vi "communication manager.vi"() -> ()   [LabVIEW 2018]
uses:
  communication-manager/socket REP/socket REP.lvclass
  C:/Users/Denis/Desktop/S4ACS/S4ACS/communication-manager/Socket/Socket.lvclass
  communication-manager/socket SUB/socket SUB.lvclass
  communication-manager/socket PUB/socket PUB.lvclass
  communication-manager/RxTx/CM_RxTx.lvclass
  <vilib>/addons/zeromq/zmq_context.lvclass
  communication-manager/Socket/Socket.lvclass
panel:
  out "error out":errorcluster
  in  "socket PUB.lvclass":refnum<class "socket PUB.lvclass">
  in  "socket SUB.lvclass":refnum<class "socket SUB.lvclass">
  in  "socket REP.lvclass":refnum<class "socket REP.lvclass">
  # "Communication Manager of S4CCS"
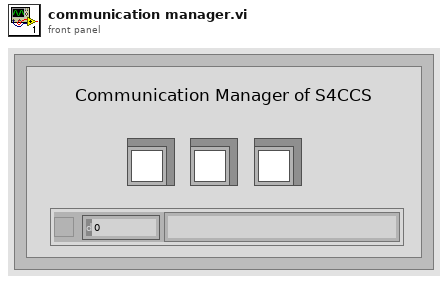
[diagram p1: front panel]
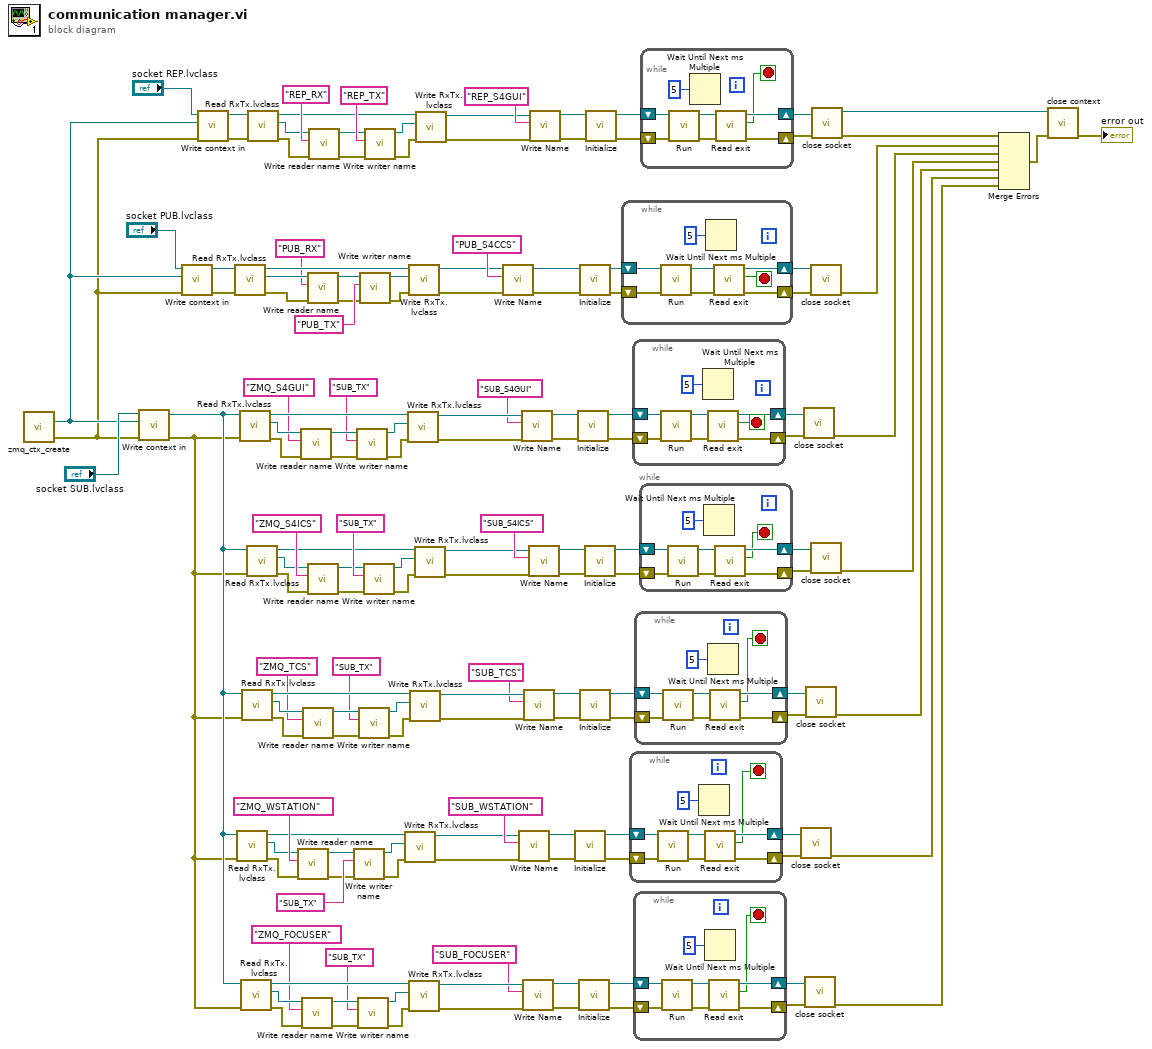
[diagram p0: block diagram]
diagram:
  n1 = call <vilib>:"zmq_ctx_create.vi"() -> ("error out"=w2:errorcluster, "context out"=w5:refnum<class "zmq_context.lvclass">)  [unwired: 4 in]
  n2 = call-dynamic "Write context in.vi"("error in (no error)"=w2, "zeromq.lvlib:ZeroMQ Context"=w5, "Socket in"="socket SUB.lvclass") -> ("error out"=w3:errorcluster, "Socket out"=w4:refnum<class "socket SUB.lvclass">)  [unwired: 7 in]
  n3 = call-dynamic "Write context in.vi"("error in (no error)"=w2, "zeromq.lvlib:ZeroMQ Context"=w5, "Socket in"="socket PUB.lvclass") -> ("error out"=w8:errorcluster, "Socket out"=w9:refnum<class "socket PUB.lvclass">)  [unwired: 7 in]
  n4 = call-dynamic "Write context in.vi"("error in (no error)"=w2, "zeromq.lvlib:ZeroMQ Context"=w5, "Socket in"="socket REP.lvclass") -> ("error out"=w11:errorcluster, "Socket out"=w12:refnum<class "socket REP.lvclass">)  [unwired: 7 in]
  n5 = call-dynamic "Read RxTx.lvclass.vi"("error in (no error)"=w8, "Socket in"=w9) -> ("error out"=w117:errorcluster, "RxTx.lvclass"=w121:refnum<class "CM_RxTx.lvclass">, "Socket out"=w118:refnum<class "socket PUB.lvclass">)  [unwired: 7 in]
  n6 = call-dynamic "Read RxTx.lvclass.vi"("error in (no error)"=w3, "Socket in"=w4) -> ("error out"=w52:errorcluster, "RxTx.lvclass"=w56:refnum<class "CM_RxTx.lvclass">, "Socket out"=w53:refnum<class "socket SUB.lvclass">)  [unwired: 7 in]
  n7 = call-dynamic "Read RxTx.lvclass.vi"("error in (no error)"=w3, "Socket in"=w4) -> ("error out"=w99:errorcluster, "RxTx.lvclass"=w95:refnum<class "CM_RxTx.lvclass">, "Socket out"=w98:refnum<class "socket SUB.lvclass">)  [unwired: 7 in]
  n8 = call-dynamic "Read RxTx.lvclass.vi"("error in (no error)"=w3, "Socket in"=w4) -> ("error out"=w33:errorcluster, "RxTx.lvclass"=w29:refnum<class "CM_RxTx.lvclass">, "Socket out"=w32:refnum<class "socket SUB.lvclass">)  [unwired: 7 in]
  n9 = call-dynamic "Read RxTx.lvclass.vi"("error in (no error)"=w3, "Socket in"=w4) -> ("error out"=w65:errorcluster, "RxTx.lvclass"=w61:refnum<class "CM_RxTx.lvclass">, "Socket out"=w64:refnum<class "socket SUB.lvclass">)  [unwired: 7 in]
  n10 = call-dynamic "Read RxTx.lvclass.vi"("error in (no error)"=w3, "Socket in"=w4) -> ("error out"=w84:errorcluster, "RxTx.lvclass"=w88:refnum<class "CM_RxTx.lvclass">, "Socket out"=w85:refnum<class "socket SUB.lvclass">)  [unwired: 7 in]
  n11 = call-dynamic "Read RxTx.lvclass.vi"("error in (no error)"=w11, "Socket in"=w12) -> ("error out"=w140:errorcluster, "RxTx.lvclass"=w144:refnum<class "CM_RxTx.lvclass">, "Socket out"=w141:refnum<class "socket REP.lvclass">)  [unwired: 7 in]
  n12 = call-dynamic "Write reader name.vi"("error in (no error)"=w52, "RX name"="ZMQ_WSTATION" ("reader name"), "RxTx in"=w56) -> ("error out"=w51:errorcluster, "RxTx out"=w55:refnum<class "CM_RxTx.lvclass">)  [unwired: 7 in]
  n13 = call-dynamic "Write reader name.vi"("error in (no error)"=w99, "RX name"="ZMQ_S4GUI" ("reader name"), "RxTx in"=w95) -> ("error out"=w100:errorcluster, "RxTx out"=w96:refnum<class "CM_RxTx.lvclass">)  [unwired: 7 in]
  n14 = call-dynamic "Write reader name.vi"("error in (no error)"=w33, "RX name"="ZMQ_FOCUSER" ("reader name"), "RxTx in"=w29) -> ("error out"=w34:errorcluster, "RxTx out"=w30:refnum<class "CM_RxTx.lvclass">)  [unwired: 7 in]
  n15 = call-dynamic "Write reader name.vi"("error in (no error)"=w65, "RX name"="ZMQ_TCS" ("reader name"), "RxTx in"=w61) -> ("error out"=w66:errorcluster, "RxTx out"=w62:refnum<class "CM_RxTx.lvclass">)  [unwired: 7 in]
  n16 = call-dynamic "Write reader name.vi"("error in (no error)"=w117, "RX name"="PUB_RX" ("reader name"), "RxTx in"=w121) -> ("error out"=w116:errorcluster, "RxTx out"=w120:refnum<class "CM_RxTx.lvclass">)  [unwired: 7 in]
  n17 = call-dynamic "Write reader name.vi"("error in (no error)"=w84, "RX name"="ZMQ_S4ICS" ("reader name"), "RxTx in"=w88) -> ("error out"=w83:errorcluster, "RxTx out"=w87:refnum<class "CM_RxTx.lvclass">)  [unwired: 7 in]
  n18 = call-dynamic "Write reader name.vi"("error in (no error)"=w140, "RX name"="REP_RX" ("reader name"), "RxTx in"=w144) -> ("error out"=w139:errorcluster, "RxTx out"=w143:refnum<class "CM_RxTx.lvclass">)  [unwired: 7 in]
  n19 = call-dynamic "Write writer name.vi"("error in (no error)"=w51, "Tx name"="SUB_TX" ("writer name"), "RxTx in"=w55) -> ("error out"=w50:errorcluster, "RxTx out"=w54:refnum<class "CM_RxTx.lvclass">)  [unwired: 7 in]
  n20 = call-dynamic "Write writer name.vi"("error in (no error)"=w100, "Tx name"="SUB_TX" ("writer name"), "RxTx in"=w96) -> ("error out"=w101:errorcluster, "RxTx out"=w97:refnum<class "CM_RxTx.lvclass">)  [unwired: 7 in]
  n21 = call-dynamic "Write writer name.vi"("error in (no error)"=w34, "Tx name"="SUB_TX" ("writer name"), "RxTx in"=w30) -> ("error out"=w35:errorcluster, "RxTx out"=w31:refnum<class "CM_RxTx.lvclass">)  [unwired: 7 in]
  n22 = call-dynamic "Write writer name.vi"("error in (no error)"=w66, "Tx name"="SUB_TX" ("writer name"), "RxTx in"=w62) -> ("error out"=w67:errorcluster, "RxTx out"=w63:refnum<class "CM_RxTx.lvclass">)  [unwired: 7 in]
  n23 = call-dynamic "Write writer name.vi"("error in (no error)"=w116, "Tx name"="PUB_TX" ("writer name"), "RxTx in"=w120) -> ("error out"=w115:errorcluster, "RxTx out"=w119:refnum<class "CM_RxTx.lvclass">)  [unwired: 7 in]
  n24 = call-dynamic "Write writer name.vi"("error in (no error)"=w83, "Tx name"="SUB_TX" ("writer name"), "RxTx in"=w87) -> ("error out"=w82:errorcluster, "RxTx out"=w86:refnum<class "CM_RxTx.lvclass">)  [unwired: 7 in]
  n25 = call-dynamic "Write writer name.vi"("error in (no error)"=w139, "Tx name"="REP_TX" ("writer name"), "RxTx in"=w143) -> ("error out"=w138:errorcluster, "RxTx out"=w142:refnum<class "CM_RxTx.lvclass">)  [unwired: 7 in]
  n26 = call-dynamic "Write RxTx.lvclass.vi"("error in (no error)"=w50, "RxTx.lvclass"=w54, "Socket in"=w53) -> ("error out"=w47:errorcluster, "Socket out"=w48:refnum<class "socket SUB.lvclass">)  [unwired: 7 in]
  n27 = call-dynamic "Write RxTx.lvclass.vi"("error in (no error)"=w101, "RxTx.lvclass"=w97, "Socket in"=w98) -> ("error out"=w104:errorcluster, "Socket out"=w103:refnum<class "socket SUB.lvclass">)  [unwired: 7 in]
  n28 = call-dynamic "Write RxTx.lvclass.vi"("error in (no error)"=w115, "RxTx.lvclass"=w119, "Socket in"=w118) -> ("error out"=w13:errorcluster, "Socket out"=w14:refnum<class "socket PUB.lvclass">)  [unwired: 7 in]
  n29 = call-dynamic "Write RxTx.lvclass.vi"("error in (no error)"=w35, "RxTx.lvclass"=w31, "Socket in"=w32) -> ("error out"=w38:errorcluster, "Socket out"=w37:refnum<class "socket SUB.lvclass">)  [unwired: 7 in]
  n30 = call-dynamic "Write RxTx.lvclass.vi"("error in (no error)"=w67, "RxTx.lvclass"=w63, "Socket in"=w64) -> ("error out"=w70:errorcluster, "Socket out"=w69:refnum<class "socket SUB.lvclass">)  [unwired: 7 in]
  n31 = call-dynamic "Write RxTx.lvclass.vi"("error in (no error)"=w82, "RxTx.lvclass"=w86, "Socket in"=w85) -> ("error out"=w79:errorcluster, "Socket out"=w80:refnum<class "socket SUB.lvclass">)  [unwired: 7 in]
  n32 = call-dynamic "Write RxTx.lvclass.vi"("error in (no error)"=w138, "RxTx.lvclass"=w142, "Socket in"=w141) -> ("error out"=w135:errorcluster, "Socket out"=w136:refnum<class "socket REP.lvclass">)  [unwired: 7 in]
  n33 = call-dynamic "Write Name.vi"("error in (no error)"=w13, "Name"="PUB_S4CCS", "Socket in"=w14) -> ("error out"=w113:errorcluster, "Socket out"=w114:refnum<class "socket PUB.lvclass">)  [unwired: 7 in]
  n34 = call-dynamic "Write Name.vi"("error in (no error)"=w47, "Name"="SUB_WSTATION", "Socket in"=w48) -> ("error out"=w21:errorcluster, "Socket out"=w22:refnum<class "socket SUB.lvclass">)  [unwired: 7 in]
  n35 = call-dynamic "Write Name.vi"("error in (no error)"=w104, "Name"="SUB_S4GUI", "Socket in"=w103) -> ("error out"=w19:errorcluster, "Socket out"=w20:refnum<class "socket SUB.lvclass">)  [unwired: 7 in]
  n36 = call-dynamic "Write Name.vi"("error in (no error)"=w38, "Name"="SUB_FOCUSER", "Socket in"=w37) -> ("error out"=w15:errorcluster, "Socket out"=w16:refnum<class "socket SUB.lvclass">)  [unwired: 7 in]
  n37 = call-dynamic "Write Name.vi"("error in (no error)"=w70, "Name"="SUB_TCS", "Socket in"=w69) -> ("error out"=w25:errorcluster, "Socket out"=w26:refnum<class "socket SUB.lvclass">)  [unwired: 7 in]
  n38 = call-dynamic "Write Name.vi"("error in (no error)"=w79, "Name"="SUB_S4ICS", "Socket in"=w80) -> ("error out"=w23:errorcluster, "Socket out"=w24:refnum<class "socket SUB.lvclass">)  [unwired: 7 in]
  n39 = call-dynamic "Write Name.vi"("error in (no error)"=w135, "Name"="REP_S4GUI", "Socket in"=w136) -> ("error out"=w17:errorcluster, "Socket out"=w18:refnum<class "socket REP.lvclass">)  [unwired: 7 in]
  n40 = call-dynamic "Initialize.vi"("error in (no error)"=w21, "socket SUB in"=w22) -> ("error out"=w44:errorcluster, "socket SUB out"=w46:refnum<class "socket SUB.lvclass">)  [unwired: 8 in]
  n41 = call-dynamic "Initialize.vi"("error in (no error)"=w19, "socket SUB in"=w20) -> ("error out"=w107:errorcluster, "socket SUB out"=w105:refnum<class "socket SUB.lvclass">)  [unwired: 8 in]
  n42 = call-dynamic "Initialize.vi"("error in (no error)"=w15, "socket SUB in"=w16) -> ("error out"=w41:errorcluster, "socket SUB out"=w39:refnum<class "socket SUB.lvclass">)  [unwired: 8 in]
  n43 = call-dynamic "Initialize.vi"("error in (no error)"=w113, "socket PUB in"=w114) -> ("error out"=w110:errorcluster, "socket PUB out"=w112:refnum<class "socket PUB.lvclass">)  [unwired: 8 in]
  n44 = call-dynamic "Initialize.vi"("error in (no error)"=w25, "socket SUB in"=w26) -> ("error out"=w73:errorcluster, "socket SUB out"=w71:refnum<class "socket SUB.lvclass">)  [unwired: 8 in]
  n45 = call-dynamic "Initialize.vi"("error in (no error)"=w23, "socket SUB in"=w24) -> ("error out"=w76:errorcluster, "socket SUB out"=w78:refnum<class "socket SUB.lvclass">)  [unwired: 8 in]
  n46 = call-dynamic "Initialize.vi"("error in (no error)"=w17, "socket REP in"=w18) -> ("error out"=w1:errorcluster, "socket REP out"=w134:refnum<class "socket REP.lvclass">)  [unwired: 8 in]
  n47 = while {
    shift-right: [w151] -> w111
    shift-left: w112 -> [w155]
    shift-right: [w150] -> w109
    shift-left: w110 -> [w154]
    stop <- w149 stop-if-true
    n48 = call-dynamic "Run.vi"("error in (no error)"=w154, "socket PUB in"=w155) -> ("error out"=w153:errorcluster, "socket PUB out"=w152:refnum<class "socket PUB.lvclass">)  [unwired: 8 in]
    n49 = Wait Until Next ms Multiple(millisecond multiple=u32 5) -> ()  [unwired: 1 out]
    n50 = call-dynamic "Read exit.vi"("error in (no error)"=w153, "Socket in"=w152) -> ("error out"=w150:errorcluster, "exit"=w149:bool, "Socket out"=w151:refnum<class "socket PUB.lvclass">)  [unwired: 7 in]
  }
  n51 = while {
    shift-right: [w161] -> w45
    shift-left: w46 -> [w163]
    shift-right: [w158] -> w43
    shift-left: w44 -> [w160]
    stop <- w157 stop-if-true
    n52 = call-dynamic "Run.vi"("error in (no error)"=w160, "socket SUB in"=w163) -> ("error out"=w159:errorcluster, "socket SUB out"=w162:refnum<class "socket SUB.lvclass">)  [unwired: 8 in]
    n53 = Wait Until Next ms Multiple(millisecond multiple=u32 5) -> ()  [unwired: 1 out]
    n54 = call-dynamic "Read exit.vi"("error in (no error)"=w159, "Socket in"=w162) -> ("error out"=w158:errorcluster, "exit"=w157:bool, "Socket out"=w161:refnum<class "socket SUB.lvclass">)  [unwired: 7 in]
  }
  n55 = while {
    shift-right: [w169] -> w106
    shift-left: w105 -> [w171]
    shift-right: [w166] -> w108
    shift-left: w107 -> [w168]
    stop <- w165 stop-if-true
    n56 = call-dynamic "Run.vi"("error in (no error)"=w168, "socket SUB in"=w171) -> ("error out"=w167:errorcluster, "socket SUB out"=w170:refnum<class "socket SUB.lvclass">)  [unwired: 8 in]
    n57 = Wait Until Next ms Multiple(millisecond multiple=u32 5) -> ()  [unwired: 1 out]
    n58 = call-dynamic "Read exit.vi"("error in (no error)"=w167, "Socket in"=w170) -> ("error out"=w166:errorcluster, "exit"=w165:bool, "Socket out"=w169:refnum<class "socket SUB.lvclass">)  [unwired: 7 in]
  }
  n59 = while {
    shift-right: [w177] -> w40
    shift-left: w39 -> [w179]
    shift-right: [w174] -> w42
    shift-left: w41 -> [w176]
    stop <- w173 stop-if-true
    n60 = call-dynamic "Run.vi"("error in (no error)"=w176, "socket SUB in"=w179) -> ("error out"=w175:errorcluster, "socket SUB out"=w178:refnum<class "socket SUB.lvclass">)  [unwired: 8 in]
    n61 = Wait Until Next ms Multiple(millisecond multiple=u32 5) -> ()  [unwired: 1 out]
    n62 = call-dynamic "Read exit.vi"("error in (no error)"=w175, "Socket in"=w178) -> ("error out"=w174:errorcluster, "exit"=w173:bool, "Socket out"=w177:refnum<class "socket SUB.lvclass">)  [unwired: 7 in]
  }
  n63 = while {
    shift-right: [w185] -> w72
    shift-left: w71 -> [w187]
    shift-right: [w182] -> w74
    shift-left: w73 -> [w184]
    stop <- w181 stop-if-true
    n64 = call-dynamic "Run.vi"("error in (no error)"=w184, "socket SUB in"=w187) -> ("error out"=w183:errorcluster, "socket SUB out"=w186:refnum<class "socket SUB.lvclass">)  [unwired: 8 in]
    n65 = Wait Until Next ms Multiple(millisecond multiple=u32 5) -> ()  [unwired: 1 out]
    n66 = call-dynamic "Read exit.vi"("error in (no error)"=w183, "Socket in"=w186) -> ("error out"=w182:errorcluster, "exit"=w181:bool, "Socket out"=w185:refnum<class "socket SUB.lvclass">)  [unwired: 7 in]
  }
  n67 = while {
    shift-right: [w193] -> w77
    shift-left: w78 -> [w195]
    shift-right: [w190] -> w75
    shift-left: w76 -> [w192]
    stop <- w189 stop-if-true
    n68 = call-dynamic "Run.vi"("error in (no error)"=w192, "socket SUB in"=w195) -> ("error out"=w191:errorcluster, "socket SUB out"=w194:refnum<class "socket SUB.lvclass">)  [unwired: 8 in]
    n69 = Wait Until Next ms Multiple(millisecond multiple=u32 5) -> ()  [unwired: 1 out]
    n70 = call-dynamic "Read exit.vi"("error in (no error)"=w191, "Socket in"=w194) -> ("error out"=w190:errorcluster, "exit"=w189:bool, "Socket out"=w193:refnum<class "socket SUB.lvclass">)  [unwired: 7 in]
  }
  n71 = while {
    shift-right: [w201] -> w133
    shift-left: w134 -> [w203]
    shift-right: [w198] -> w132
    shift-left: w1 -> [w200]
    stop <- w197 stop-if-true
    n72 = call-dynamic "Run.vi"("error in (no error)"=w200, "socket REP in"=w203) -> ("error out"=w199:errorcluster, "socket REP out"=w202:refnum<class "socket REP.lvclass">)  [unwired: 8 in]
    n73 = Wait Until Next ms Multiple(millisecond multiple=u32 5) -> ()  [unwired: 1 out]
    n74 = call-dynamic "Read exit.vi"("error in (no error)"=w199, "Socket in"=w202) -> ("error out"=w198:errorcluster, "exit"=w197:bool, "Socket out"=w201:refnum<class "socket REP.lvclass">)  [unwired: 7 in]
  }
  n75 = call "close socket.vi"("error in (no error)"=w43, "Socket in"=w45) -> ("error out"=w123:errorcluster)  [unwired: 8 in, 1 out]
  n76 = call "close socket.vi"("error in (no error)"=w108, "Socket in"=w106) -> ("error out"=w129:errorcluster)  [unwired: 8 in, 1 out]
  n77 = call "close socket.vi"("error in (no error)"=w42, "Socket in"=w40) -> ("error out"=w122:errorcluster)  [unwired: 8 in, 1 out]
  n78 = call "close socket.vi"("error in (no error)"=w74, "Socket in"=w72) -> ("error out"=w124:errorcluster)  [unwired: 8 in, 1 out]
  n79 = call "close socket.vi"("error in (no error)"=w109, "Socket in"=w111) -> ("error out"=w130:errorcluster)  [unwired: 8 in, 1 out]
  n80 = call "close socket.vi"("error in (no error)"=w75, "Socket in"=w77) -> ("error out"=w125:errorcluster)  [unwired: 8 in, 1 out]
  n81 = call "close socket.vi"("error in (no error)"=w132, "Socket in"=w133) -> ("error out"=w131:errorcluster, "Socket out"=w127:refnum<class "socket REP.lvclass">)  [unwired: 8 in]
  n82 = Merge Errors(w131, w130, w129, w125, w124, w123, w122) -> (w128:errorcluster)
  n83 = call-dynamic "close context.vi"("error in (no error)"=w128, "Socket in"=w127) -> ("error out"=→"error out":errorcluster)  [unwired: 8 in, 1 out]
